vi "from string 1.0.vi"(8 "error in (no error)":errorcluster, 10 "data":string, 11 "PID Module  configuration in":refnum<class "PID Module configuration.lvclass">) -> (0 "error out":errorcluster, 3 "PID Module  configuration out":refnum<class "PID Module configuration.lvclass">)   [LabVIEW 2015, in "PID Module configuration.lvclass"]
uses:
  PID Module configuration.lvclass
  PID Module configuration.lvclass/PID Module configuration.ctl
  <vilib>/NI/Tag Bus/tag/default value polymorphs/write default value Double.vi
  <vilib>/NI/Configuration Framework/serializable configuration/NISE_CEF_serializable configuration.lvclass
  <vilib>/NI/Tag Bus/tag/tag descriptor.lvclass
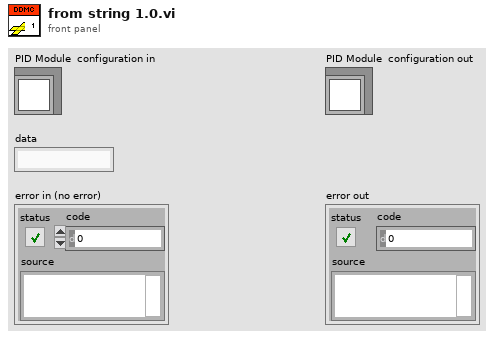
[diagram p1: front panel]
types:
  T1 = typedef "PID Module configuration.lvclass/Line.ctl" = cluster{"PID ID":string, "Setpoint":refnum<class "TBM channel.lvclass">, "Variable":refnum<class "TBM channel.lvclass">, "Output":refnum<class "TBM channel.lvclass">, "Output High":refnum<class "TBM channel.lvclass">, "Output Low":refnum<class "TBM channel.lvclass">, "P":refnum<class "TBM channel.lvclass">, "I":refnum<class "TBM channel.lvclass">, "D":refnum<class "TBM channel.lvclass">}
  T2 = typedef "PID Module configuration.lvclass/PID Range.ctl" = cluster{"output high":dbl, "output low":dbl}
  T3 = typedef "PID Module configuration.lvclass/PID Gains.ctl" = cluster{"proportional gain (Kc)":dbl, "integral time (Ti, min)":dbl, "derivative time (Td, min)":dbl}
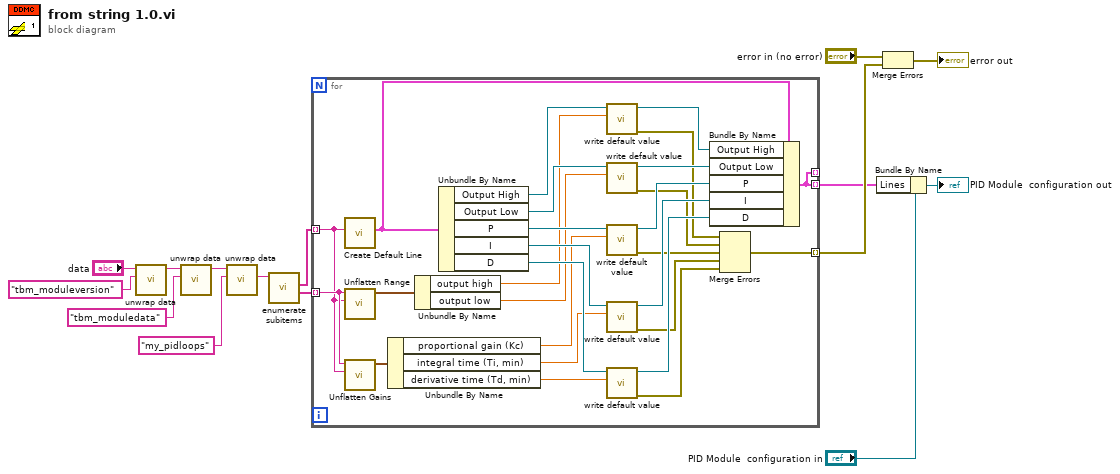
[diagram p0: block diagram]
diagram:
  n1 = call <vilib>:"unwrap data.vi"("identifier"="tbm_moduleversion" ("additional identifier"), "data to unwrap"="data") -> ("remaining string"=w10:string)  [unwired: 8 in, 1 out]
  n2 = call <vilib>:"unwrap data.vi"("identifier"="tbm_moduledata" ("additional identifier"), "data to unwrap"=w10) -> ("remaining string"=w8:string)  [unwired: 8 in, 1 out]
  n3 = call <vilib>:"unwrap data.vi"("identifier"="my_pidloops" ("additional identifier"), "data to unwrap"=w8) -> ("unwrapped data"=w6:string)  [unwired: 8 in, 1 out]
  n4 = call <vilib>:"enumerate subitems.vi"("data to enumerate"=w6) -> ("associated data"=w3:string[], "discovered subitems"=w4:string[])  [unwired: 8 in, 1 out]
  n5 = for {
    tunnel: [w42] -> w12 mode=indexing
    tunnel: w4 -> [w20] mode=indexing
    tunnel: w3 -> [w21] mode=indexing
    tunnel: [w16] -> _ mode=indexing
    tunnel: [w16] -> w1 mode=indexing
    n6 = call "Create Default Line.vi"("Line Name"=w20) -> ("Default Line"=w41:T1)  [unwired: 10 in]
    n7 = call "Unflatten Range.vi"("Identifier"=w20, "Data to Unwrap"=w21) -> ("output range"=w25:T2)  [unwired: 9 in]
    n8 = call "Unflatten Gains.vi"("Identifier"=w20, "Data to Unwrap"=w21) -> ("PID gains"=w22:T3)  [unwired: 9 in]
    n9 = Unbundle By Name(w22) -> ("proportional gain (Kc)"=w19:dbl, "integral time (Ti, min)"=w18:dbl, "derivative time (Td, min)"=w17:dbl)
    n10 = Unbundle By Name(w25) -> ("output high"=w24:dbl, "output low"=w23:dbl)
    n11 = Unbundle By Name(w41) -> ("Output High"=w40:refnum<class "TBM channel.lvclass">, "Output Low"=w38:refnum<class "TBM channel.lvclass">, "P"=w36:refnum<class "TBM channel.lvclass">, "I"=w35:refnum<class "TBM channel.lvclass">, "D"=w34:refnum<class "TBM channel.lvclass">)
    n12 = call-poly <vilib>:"write default value.vi"("default value"=w24, "system tag in"=w40) -> ("error out"=w30:errorcluster, "system tag out"=w39:refnum<class "TBM channel.lvclass">)  [unwired: 8 in]
    n13 = call-poly <vilib>:"write default value.vi"("default value"=w23, "system tag in"=w38) -> ("error out"=w29:errorcluster, "system tag out"=w37:refnum<class "TBM channel.lvclass">)  [unwired: 8 in]
    n14 = call-poly <vilib>:"write default value.vi"("default value"=w19, "system tag in"=w36) -> ("error out"=w28:errorcluster, "system tag out"=w33:refnum<class "TBM channel.lvclass">)  [unwired: 8 in]
    n15 = call-poly <vilib>:"write default value.vi"("default value"=w18, "system tag in"=w35) -> ("error out"=w27:errorcluster, "system tag out"=w32:refnum<class "TBM channel.lvclass">)  [unwired: 8 in]
    n16 = call-poly <vilib>:"write default value.vi"("default value"=w17, "system tag in"=w34) -> ("error out"=w26:errorcluster, "system tag out"=w31:refnum<class "TBM channel.lvclass">)  [unwired: 8 in]
    n17 = Bundle By Name(cluster=w41, "Output High"=w39, "Output Low"=w37, "P"=w33, "I"=w32, "D"=w31) -> (w16:T1)
    n18 = Merge Errors(w30, w29, w28, w27, w26) -> (w42:errorcluster)
  }
  n19 = Bundle By Name(cluster="PID Module  configuration in", "Lines"=w1) -> (→"PID Module  configuration out":refnum<class "PID Module configuration.lvclass">)
  n20 = Merge Errors("error in (no error)", w12) -> (→"error out":errorcluster)
